vi "cluster_v06.vi"() -> ()   [LabVIEW 2009]
panel:
  in  "stop":bool
  in  "Slide":u8(slide)=8 scale=0.0..10.0
  out "XY Graph":cluster{dbl[], dbl[]}(graph)={[0.6932260777775765, -0.3679086452937484, 0.23257179032719136, -0.9443331009843002, -0.10671015871737696, -0.37766465858981596, 0.10336049429117579, 0.6630395530323785, 0.09424591796811296, 0.8112228801529898, -0.49649174526535356, 0.06992954088535386, -0.7425130982768668, -0.3693301461468815, 0.03552789351925686, -0.12372967395565591, 0.9241198265489284, -0.024938719206913696, 0.7021054343819679, -0.4062911427719912, -0.26361410960415016, -0.41669590674450346, -0.6403934450987672, 0.379034631718192, -0.20330930604893707, 0.9653743910826671, 0.06563933538821022, 0.3859826097158176, -0.17256023496973166, -0.6431869956433118, -0.11376808087234225, -0.7767996723116578, 0.534029129468839, -0.06971186789894446, 0.7792056505051659, 0.3117276233700289, -0.02758845092143779, 0.06641282796769997, -0.9187396644286306, 0.03550201397484128, -0.6913206643994623, 0.46642208124923845, 0.2440665508991571, 0.45384277288355734, 0.5844050824739737, -0.3876413789490265, 0.17202464545129278, -0.981512243080157, -0.025258692200358226, -0.39230101095832876, 0.24109547848074345, 0.6203518753363269, 0.13379275180192568, 0.7381980513286116, -0.5682745231606543, 0.06815972048752823, -0.8122060164063085, -0.25314057380837224, 0.019227386096682467, -0.008053911446189046, 0.9087148301607435, -0.0446776436911911, 0.6767210560969622], [0.06955461119489617, -0.7228520638261612, -0.39766207166806006, 0.03929998447744605, -0.1519047369600601, 0.9250478173902662, -0.019148795737514858, 0.7060662628760096, -0.3753247784801221, -0.2731391708019039, -0.3975852786052707, -0.6672223411686191, 0.37378733499680034, -0.21820127445575618, 0.9554601944106752, 0.08610243053103847, 0.3820660534389099, -0.13802063465079745, -0.6534967943584111, -0.10393537155242147, -0.7945439914745376, 0.5156623729759519, -0.06998436390060844, 0.7613072178914418, 0.3406720279321079, -0.03161884288545853, 0.09522017728825255, -0.9220147901561087, 0.0303916116907844, -0.6971904453411177, 0.4366698015271052, 0.2539161342961245, 0.43545852214383574, 0.6127753579492323, -0.38365186185975747, 0.1879115490042415, -0.9740623151179858, -0.04534892017404063, -0.38939910713517384, 0.20693367090791132, 0.6321313262423321, 0.12372654053858007, 0.7580103803795478, -0.5515725675368365, 0.06910556735513591, -0.7961807453901462, -0.2825370490654184, 0.023452596773614852, -0.03734482038013741, 0.9143029809952036, -0.04026529256236226, 0.6844968297315264, -0.4955102384369383, -0.23408666487533372, -0.4718186074345754, -0.5553206036352875, 0.39100655061794315, -0.15566619682191696, 0.9877141206002635, 0.005395580061316444, 0.39467450379781377, -0.275000417481818, -0.6078716125232543]}
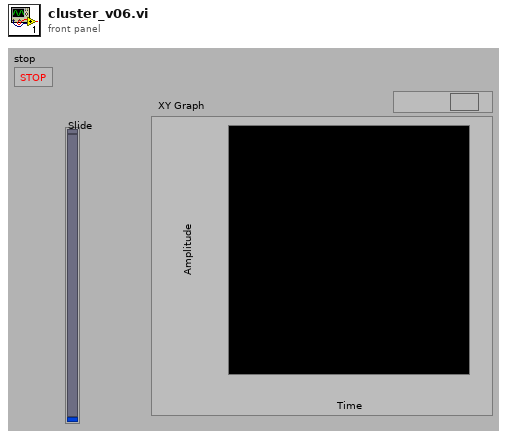
[diagram p1: front panel]
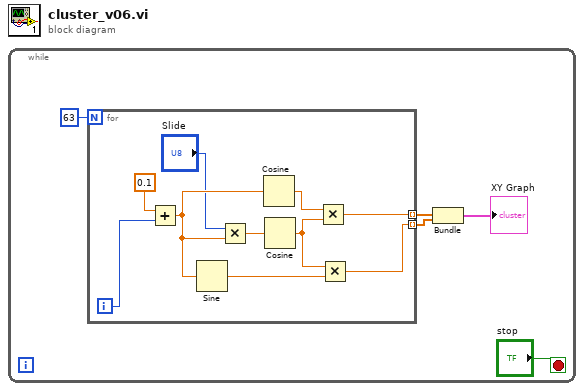
[diagram p0: block diagram]
diagram:
  n1 = while {
    stop <- "stop" stop-if-true
    n2 = for {
      N: 63 -> [_]
      tunnel: [w11] -> w4 mode=indexing
      tunnel: [w7] -> w3 mode=indexing
      i -> [w15]
      n3 = Add(x=0.1, y=w15) -> (x+y=w10:dbl)
      n4 = Sine(x=w10) -> (sin(x)=w8:dbl)
      n5 = Multiply(x="Slide", y=w10) -> (x*y=w13:dbl)
      n6 = Cosine(x=w10) -> (cos(x)=w12:dbl)
      n7 = Cosine(x=w13) -> (cos(x)=w9:dbl)
      n8 = Multiply(x=w12, y=w9) -> (x*y=w11:dbl)
      n9 = Multiply(x=w9, y=w8) -> (x*y=w7:dbl)
    }
    n10 = Bundle(w4, w3) -> (→"XY Graph":cluster{dbl[], dbl[]})  [unwired: 1 in]
  }
